vi "start.vi"(8 "error in (no error)":errorcluster, 11 "DataCollectionDL110128Streaming in":refnum<class "DataCollectionDL110128Streaming.lvclass">) -> (0 "error out":errorcluster, 3 "DataCollectionDL110128Streaming out":refnum<class "DataCollectionDL110128Streaming.lvclass">)   [LabVIEW 2010, in "DataCollectionDL110128Streaming.lvclass"]
uses:
  DataCollectionDL110128Streaming.lvclass
  DataCollectionDL110128Streaming.lvclass/DataCollectionDL110128Streaming.ctl
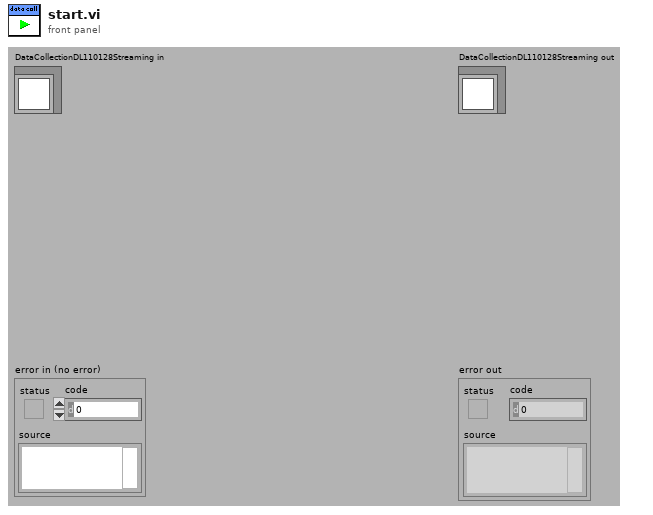
[diagram p1: front panel]
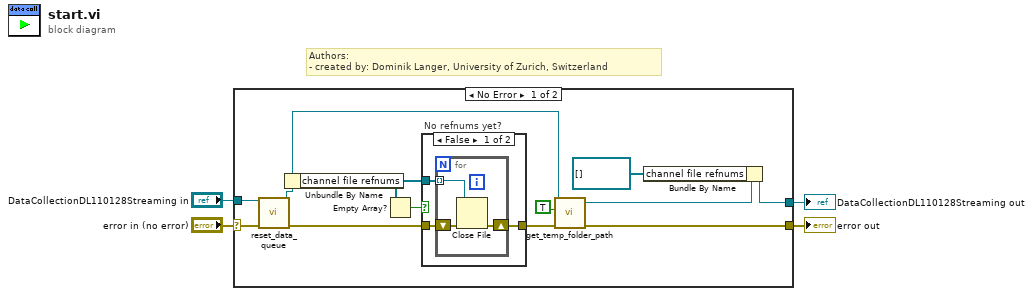
[diagram p0: block diagram]
diagram:
  # "Authors: \n- created by: Dominik Langer, University of Zurich, Switzerland"
  n1 = case shown="No Error" "error in (no error)" {
    selector: "error in (no error)" -> [w15 w25]
    tunnel: [w9 w25] -> w3
    tunnel: [w6 w24] -> w1
    tunnel: "DataCollectionDL110128Streaming in" -> [w16 w24]
    frame No Error {
      n2 = call-dynamic "reset_data_queue.vi"("error in (no error)"=w15, "GenericToplevelComponent in"=w16) -> ("error out"=w14:errorcluster, "GenericToplevelComponent out"=w8:refnum<class "DataCollectionDL110128Streaming.lvclass">)  [unwired: 8 in]
      n3 = Unbundle By Name(w8) -> ("channel file refnums"=w10:refnum<file>[])
      n4 = Empty Array?(array=w10) -> (empty?=w11:bool)
      n5 = case "No refnums yet?" shown="False" w11 {
        tunnel: w14 -> [w19 w23]
        tunnel: [w17 w23] -> w12
        tunnel: w10 -> [w18 _]
        frame False {
          n6 = for {
            tunnel: w18 -> [w21] mode=indexing
            shift-right: [w20] -> w17
            shift-left: w19 -> [w22]
            n7 = Close File(refnum=w21, error in=w22) -> (error out=w20:errorcluster)  [unwired: 1 out]
          }
        }
        frame True {
        }
      }
      n8 = call-dynamic "get_temp_folder_path.vi"("error in (no error)"=w12, "flush?"=TRUE, "GenericComponent in"=w8) -> ("error out"=w9:errorcluster, "GenericComponent out"=w7:refnum<class "DataCollectionDL110128Streaming.lvclass">)  [unwired: 6 in, 1 out]
      n9 = Bundle By Name(cluster=w7, "channel file refnums"=refnum<file>[] []) -> (w6:refnum<class "DataCollectionDL110128Streaming.lvclass">)
    }
    frame Error {
    }
  }
  "error out" <- w3
  "DataCollectionDL110128Streaming out" <- w1
